vi "CH_LM Config Statistics Batch Size.vi"(0 "Meter Index":i32, 2 "Batch Size (2)":i32=2, 3 "Sample Rate (1)":i32=1, 5 "error in (no error)":errorcluster, 7 "Timeout / ms (3000)":i32=3000, 8 "Action (query)":bool, 9 "Lock Timeout / ms (1000)":i32=1000) -> (11 "Lock timed out":bool, 14 "Meter Index":i32, 16 "Batch Size":i32, 17 "Sample Rate":i32, 19 "error out":errorcluster)   [LabVIEW 2012, in "CH_LM.lvlib"]
doc: "This command will set/query the statistics batch size and statistics sampling rate, which takes effect at the end of the current statistical batch.\n\nMeasurement data will be added to the batch on a sub-sampled basis ranging from as low as 1 pulse added per 99999 measured to as high as 1 pulse added per 1 measured. The statistics sampling rate will indicate the number of pulses that will be measured for every one pulse added to the batch.\n\n<B>Attention:</B> This command will apply only under one of the following conditions:\n- a pyroelectric probe is attached \n- a thermopile probe is attached and Joules mode is selected"
uses:
  CH_LM.lvlib
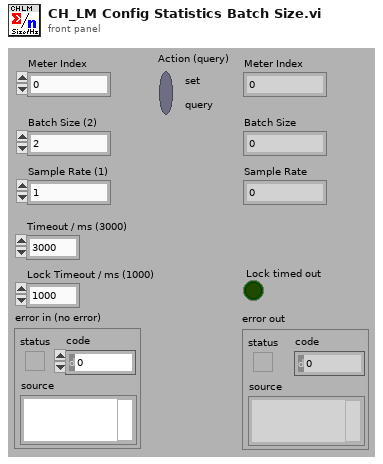
[diagram p1: front panel]
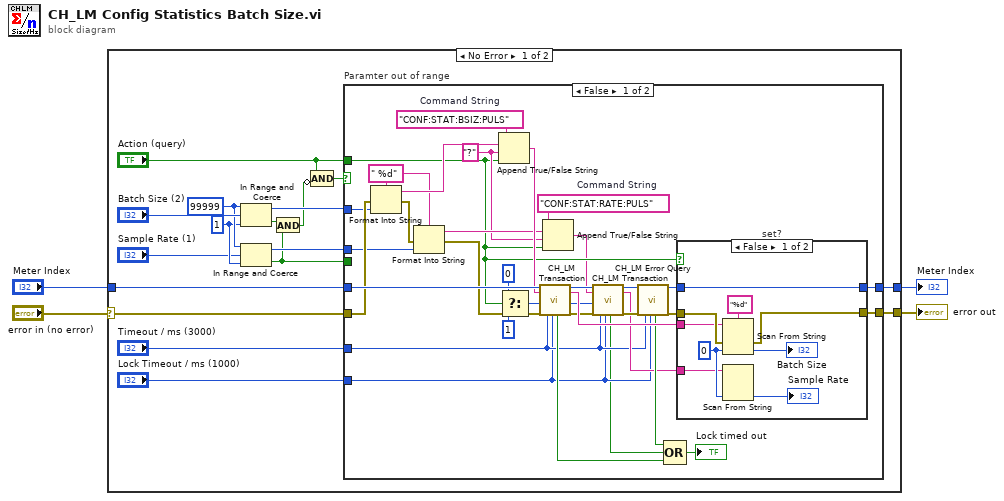
[diagram p0: block diagram]
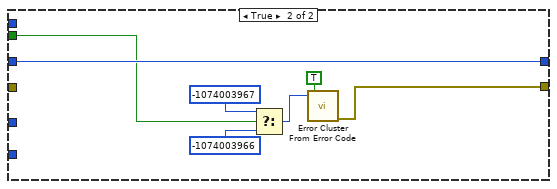
[diagram p3: hidden frame]
diagram:
  n1 = case shown="No Error" "error in (no error)" {
    selector: "error in (no error)" -> [w21 w75]
    tunnel: [w19 w75] -> w4
    tunnel: "Meter Index" -> [w20 w74]
    tunnel: [w18 w74] -> w1
    frame No Error {
      w10 = 1 ("lower limit")
      w11 = 99999 ("upper limit")
      n2 = In Range and Coerce(upper limit=w11, x="Batch Size (2)", lower limit=w10) -> (coerced(x)=w15:i32, In Range?=w9:bool)
      n3 = In Range and Coerce(upper limit=w11, x="Sample Rate (1)", lower limit=w10) -> (coerced(x)=w7:i32, In Range?=w6:bool)
      n4 = And(x=w9, y=w6) -> (x .and. y?=w8:bool)
      n5 = Compound Arithmetic op=AND("Action (query)", invert w8) -> (w13:bool)
      n6 = case "Paramter out of range" shown="False" w13 {
        tunnel: w21 -> [w43 _]
        tunnel: w20 -> [w55 w73]
        tunnel: [w52 w71] -> w19
        tunnel: [w49 w73] -> w18
        tunnel: "Timeout / ms (3000)" -> [w24 _]
        tunnel: "Lock Timeout / ms (1000)" -> [w23 _]
        tunnel: w15 -> [w40 _]
        tunnel: "Action (query)" -> [w28 _]
        tunnel: w7 -> [w32 _]
        tunnel: w6 -> [_ w68]
        frame False {
          w25 = "CONF:STAT:RATE:PULS"  # Command String
          w31 = " %d" ("format string")
          w29 = "?" ("true string")
          w54 = "CONF:STAT:BSIZ:PULS"  # Command String
          n7 = Format Into String(format string=w31, error in=w43, w40) -> (resulting string=w41:string, error out=w34:errorcluster)  [unwired: 1 in]
          n8 = Format Into String(format string=w31, error in=w34, w32) -> (resulting string=w30:string, error out=w33:errorcluster)  [unwired: 1 in]
          n9 = Append True/False String(1:w28, 2:w29, 3:w41, 4:w54) -> (0:w42:string)
          n10 = Select(t=0, s=w28, f=1 ("NofStrings (-1:all)")) -> (s? t:f=w26:i32)
          n11 = call "CH_LM Transaction.vi"("Meter Index"=w55, "Command String"=w42, "NofStrings (-1:all)"=w26, "error in (no error)"=w33, "Timeout / ms (3000)"=w24, "Lock Timeout / ms (1000)"=w23) -> ("Lock timed out"=w45:bool, "Meter Index"=w39:i32, "Response"=w53:string, "error out"=w38:errorcluster)  [unwired: 10 out]
          n12 = Append True/False String(1:w28, 2:w29, 3:w30, 4:w25) -> (0:w27:string)
          n13 = call "CH_LM Transaction.vi"("Meter Index"=w39, "Command String"=w27, "NofStrings (-1:all)"=w26, "error in (no error)"=w38, "Timeout / ms (3000)"=w24, "Lock Timeout / ms (1000)"=w23) -> ("Lock timed out"=w22:bool, "Meter Index"=w37:i32, "Response"=w35:string, "error out"=w36:errorcluster)  [unwired: 10 out]
          n14 = call "CH_LM Error Query.vi"("Meter Index"=w37, "error in (no error)"=w36, "Timeout / ms (3000)"=w24, "Lock Timeout / ms (1000)"=w23) -> ("Lock timed out"=w46:bool, "Meter Index"=w48:i32, "error out"=w47:errorcluster)  [unwired: 13 out]
          n15 = Compound Arithmetic op=OR(w46, w22, w45) -> (→"Lock timed out":bool)
          n16 = case "set?" shown="False" w28 {
            tunnel: w53 -> [w60 _]
            tunnel: w47 -> [w64 w66]
            tunnel: [w63 w66] -> w52
            tunnel: w48 -> [w62 w65]
            tunnel: [w62 w65] -> w49
            tunnel: w35 -> [w57 _]
            frame False {
              w58 = 0 ("default value 1")
              n17 = Scan From String(format string="%d", input string=w60, error in=w64, default 1=w58) -> (error out=w63:errorcluster, output 1=→"Batch Size":i32)  [unwired: 1 in, 2 out]
              n18 = Scan From String(input string=w57, default 1=w58) -> (output 1=→"Sample Rate":i32)  [unwired: 3 in, 3 out]
            }
            frame True {
            }
          }
        }
        frame True {
          n19 = Select(t=-1074003967 ("error code (0)"), s=w68, f=-1074003966 ("error code (0)")) -> (s? t:f=w69:i32)
          n20 = call <vilib>:"Error Cluster From Error Code.vi"("show call chain? (False)"=TRUE, "error code (0)"=w69) -> ("error out"=w71:errorcluster)  [unwired: 1 in, 6 out]
        }
      }
    }
    frame Error {
    }
  }
  "error out" <- w4
  "Meter Index" <- w1
